vi "FT10_Connect Fornax TCP-IP.vi"(8 "error in (no error)":errorcluster, 11 "Message Handling Cluster in":T2) -> (0 "error out":errorcluster, 1 "Array":T5(array[cluster]), 2 "Fornax Connected?":bool, 3 "Message Handling Cluster out":T2)   [LabVIEW 2024]
uses:
  Controls/Control_Message Handling Cluster.ctl
  Controls/Control_M4X Connection.ctl
  Controls/Control_PXI-7854R FPGA Reference.ctl
panel:
  out "Cluster":T1
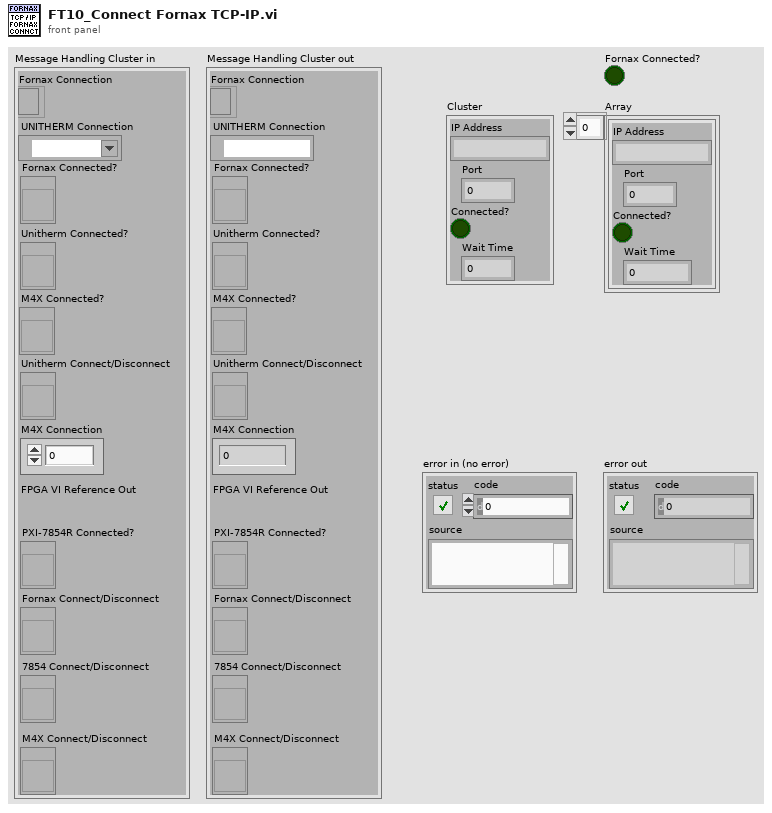
[diagram p1: front panel]
types:
  T1 = cluster{"IP Address":string, "Port":u16, "Connected?":bool, "Wait Time":dbl}
  T2 = typedef "Control_Message Handling Cluster.ctl" = cluster{"Fornax Connected?":refnum<vi>, "Unitherm Connected?":refnum<vi>, "M4X Connected?":refnum<vi>, "Unitherm Connect/Disconnect":refnum<vi>, "Fornax Connection":refnum<k5>, "UNITHERM Connection":refnum<visa-resource-name>, "M4X Connection":T3, "PXI-7854R FPGA Reference":T4, "PXI-7854R Connected?":refnum<vi>, "Fornax Connect/Disconnect":refnum<vi>, "7854 Connect/Disconnect":refnum<vi>, "M4X Connect/Disconnect":refnum<vi>}
  T3 = typedef "Control_M4X Connection.ctl" = u32
  T4 = typedef "Control_PXI-7854R FPGA Reference.ctl" = refnum<k20>
  T5 = cluster{"IP Address":string, "Port":u16, "Connected?":bool, "Wait Time":dbl}[]
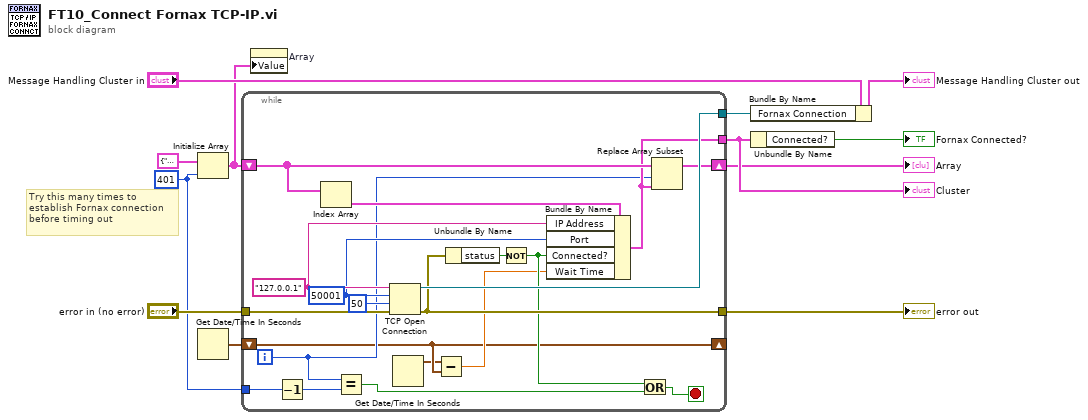
[diagram p0: block diagram]
diagram:
  w3 = 401 ("dimension size")
  # "Try this many times to \nestablish Fornax connection\nbefore timing out"
  n1 = Initialize Array(T1 {"IP Address"="", "Port"=0, "Connected?"=FALSE, "Wait Time"=0.0} ("Cluster"), w3) -> (w1:T5)
  n2 = Get Date/Time In Seconds() -> (seconds since 1Jan1904=w5:timestamp)
  n3 = while {
    tunnel: [w31] -> w12
    shift-right: [w30] -> w4
    shift-left: w1 -> [w29]
    tunnel: w3 -> [w20]
    tunnel: [w17] -> w9
    shift-right: [w14] -> _
    shift-left: w5 -> [w14]
    tunnel: "error in (no error)" -> [w32]
    tunnel: [w25] -> w7
    i -> [w16]
    stop <- w22 stop-if-true
    w26 = u16 50001 ("remote port or service name")
    w27 = "127.0.0.1" ("address")
    n4 = Decrement(x=w20) -> (x-1=w19:i32)
    n5 = Index Array(array=w29) -> (element=w28:T1)  [unwired: 1 in]
    n6 = Equal?(x=w16, y=w19) -> (x = y?=w18:bool)
    n7 = TCP Open Connection(address=w27, remote port or service name=w26, timeout ms (60000)=50, error in (no error)=w32) -> (connection ID=w31:refnum<k5>, error out=w25:errorcluster)  [unwired: 1 in]
    n8 = Get Date/Time In Seconds() -> (seconds since 1Jan1904=w13:timestamp)
    n9 = Subtract(x=w13, y=w14) -> (x-y=w15:dbl)
    n10 = Unbundle By Name(w25) -> ("status"=w24:bool)
    n11 = Not(x=w24) -> (.not. x?=w21:bool)
    n12 = Bundle By Name(cluster=w28, "IP Address"=w27, "Port"=w26, "Connected?"=w21, "Wait Time"=w15) -> (w17:T1)
    n13 = Or(x=w21, y=w18) -> (x .or. y?=w22:bool)
    n14 = Replace Array Subset(array=w29, new element=w17, index=w16) -> (w30:T5)
  }
  "Array" <- w4
  "error out" <- w7
  "Cluster" <- w9
  n15 = property on="Array" class="Arr (strict)"("Value"=w1) -> ()  [unwired: 2 in, 2 out]
  n16 = Bundle By Name(cluster="Message Handling Cluster in", "Fornax Connection"=w12) -> (→"Message Handling Cluster out":T2)
  n17 = Unbundle By Name(w9) -> ("Connected?"=→"Fornax Connected?":bool)
